vi "Write LED.vi"(6 "error in (no error)":errorcluster, 7 "VISA resource name":refnum<visa-resource-name>, 8 "B":u32, 9 "G":u32, 10 "R":u32, 11 "Index":i32) -> (0 "error out":errorcluster, 3 "VISA resource name out":refnum<visa-resource-name>)   [LabVIEW 2020]
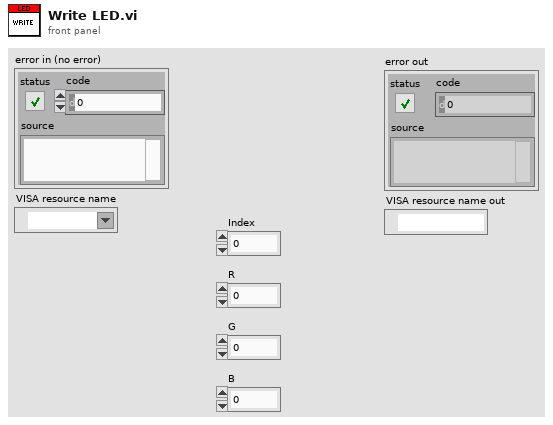
[diagram p1: front panel]
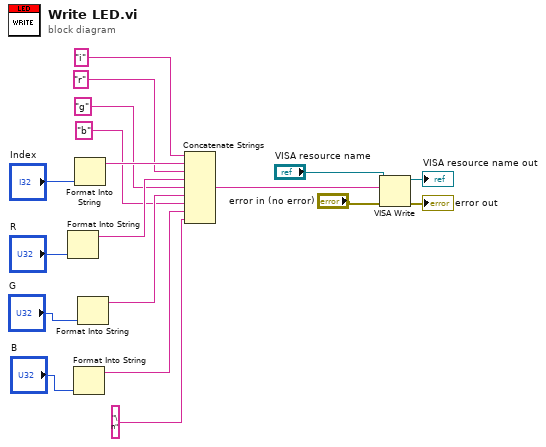
[diagram p0: block diagram]
diagram:
  n1 = Format Into String("R") -> (resulting string=w11:string)  [unwired: 3 in, 1 out]
  n2 = Format Into String("B") -> (resulting string=w7:string)  [unwired: 3 in, 1 out]
  n3 = Format Into String("Index") -> (resulting string=w16:string)  [unwired: 3 in, 1 out]
  n4 = Format Into String("G") -> (resulting string=w9:string)  [unwired: 3 in, 1 out]
  n5 = Concatenate Strings("i" ("string"), w16, "r" ("string"), w11, "g" ("string"), w9, "b" ("string"), w7, "\n" ("string")) -> (w1:string)
  n6 = VISA Write(VISA resource name="VISA resource name", write buffer=w1, error in (no error)="error in (no error)") -> (VISA resource name out=→"VISA resource name out":refnum<visa-resource-name>, error out=→"error out":errorcluster)  [unwired: 1 out]
